vi "IP Cam Loop.vi"(11 "CameraDevRef":T1) -> ()   [LabVIEW 2015]
doc: "This VI acquires the image buffer from the camera MJPG stream at the configured fps rate. It notifies any waiting VIs and allows them to pick up the latest image. This allows the camera and robot vision loop to run at different rates. The 1011, camera is far more efficient using MJPGs, and generally, this is probably the better choice for the camera loop.\n \nThis software is licensed. Open the labview\\readme\\WPI Robotics Library Open Source License.txt file for more information."
uses:
  <vilib>/Rock Robotics/WPI/Camera/WPI_CameraDevRef.ctl
  <vilib>/Rock Robotics/WPI/Camera/WPI_CameraSettings Operations.ctl
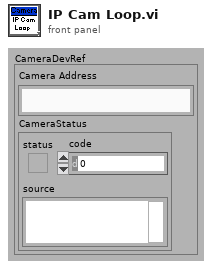
[diagram p1: front panel]
types:
  T1 = typedef "WPI_CameraDevRef.ctl" = cluster{"Camera Address":string, "CameraStatus":errorcluster}
  T2 = typedef "WPI_CameraSettings Operations.ctl" = enum16{"Udate FPS", "Update Compression", "Update Size", "Update White Balance", "Update Brightness", "Update Sharpness", "Update Exposure", "Update Exposure Value", "Update Color Level", "Update Exp Priority", "Update Color Enable", "Update JPG", "Update MJPG", "Read and Clear", "Read", "Init"}
  T3 = typedef "WPI_CameraSettings Control.ctl" = cluster{"FPS":i32, "Compression":i32, "Size":i32, "White Balance":i32, "Brightness":i32, "Sharpness":i32, "Exposure":i32, "Color Level":i32, "Exposure Priority":i32, "Color Enable":i32, "JPG Loop":i32, "MJPG Loop":i32, "Exposure Value":i32}
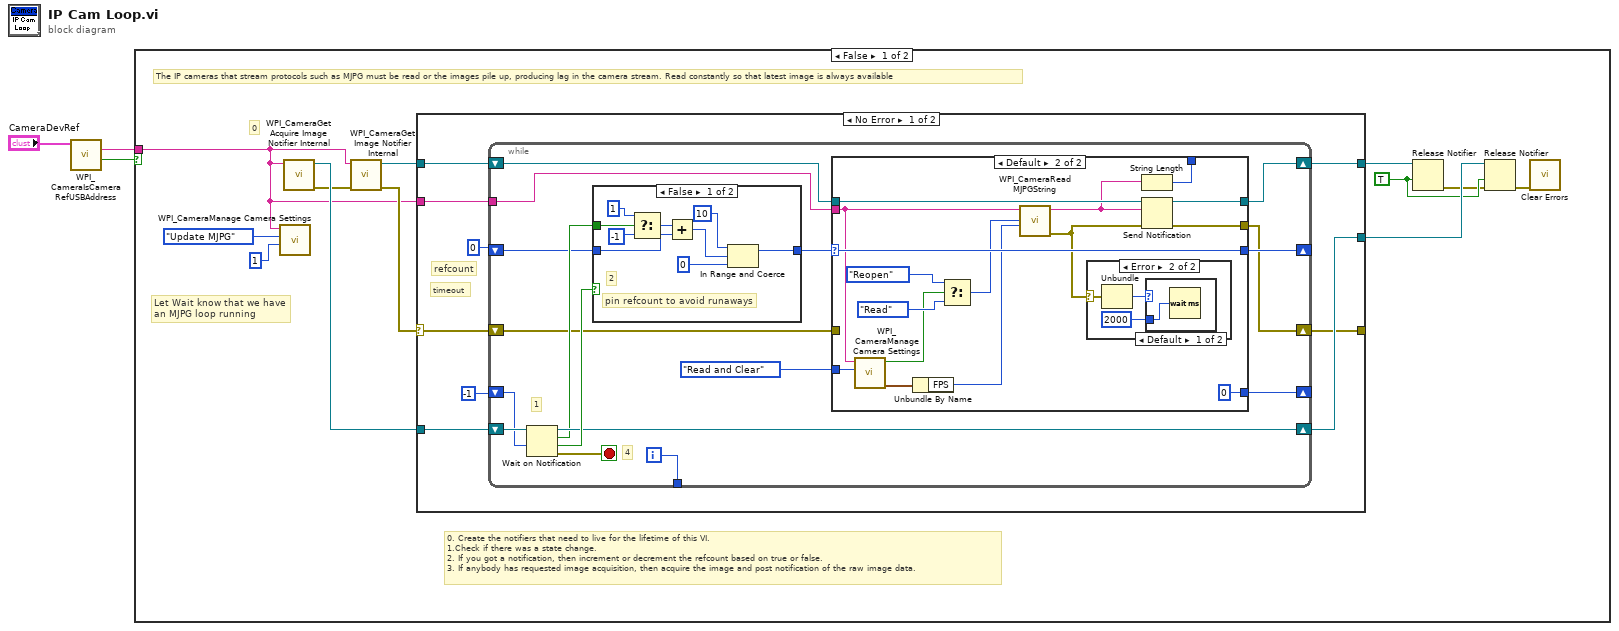
[diagram p0: block diagram]
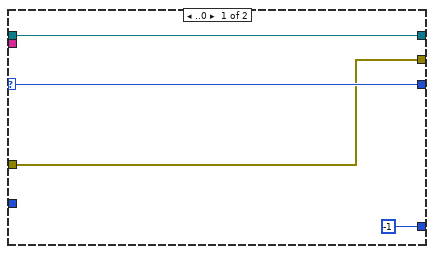
[diagram p2: hidden frame]
diagram:
  n1 = call <vilib>:"WPI_CameraIsCameraRefUSBAddress.vi"("CameraDevRef"="CameraDevRef") -> ("USB?"=w2:bool, "Camera Address Out"=w1:string)  [unwired: 7 in, 2 out]
  n2 = case shown="False" w2 {
    tunnel: w1 -> [w5 _]
    frame False {
      w12 = TRUE ("force destroy? (F)")
      # "The IP cameras that stream protocols such as MJPG must be read or the images pile up, producing lag in the camera stream. Read constantly so that latest image is always available"
      # "0. Create the notifiers that need to live for the lifetime of this VI. \n1.Check if there was a state change.\n2. If you got a notification, then increment or decrement the refcount based on true or false.\n3. If anybody has requested image acquisition, then acquire the image and post notification of the raw image data."
      # "Let Wait know that we have\nan MJPG loop running"
      # "0"
      n3 = call <vilib>:"WPI_CameraManage Camera Settings.vi"("Value"=1, "Operation"=WPI_CameraSettings_Operations."Update MJPG", "Camera IP"=w5) -> ()  [unwired: 7 in, 2 out]
      n4 = call <vilib>:"WPI_CameraGet Acquire Image Notifier Internal.vi"("Camera Address"=w5) -> ("error out"=w9:errorcluster, "Acquire Image Notifier"=w10:refnum<notifier>)  [unwired: 1 in, 8 out]
      n5 = call <vilib>:"WPI_CameraGet Image Notifier Internal.vi"("error in (no error)"=w9, "Camera Address"=w5) -> ("error out"=w11:errorcluster, "Image Notifier"=w13:refnum<notifier>)  [unwired: 8 out]
      n6 = case shown="No Error" w11 {
        selector: w11 -> [w17 w78]
        tunnel: w5 -> [w24 _]
        tunnel: w10 -> [w23 w76]
        tunnel: w13 -> [w21 w77]
        tunnel: [w19 w77] -> w15
        tunnel: [w18 w76] -> w14
        tunnel: [w16 w78] -> _
        frame No Error {
          # "timeout"
          # "refcount"
          n7 = while {
            shift-right: [w39] -> w18
            shift-left: w23 -> [w41]
            tunnel: w24 -> [w36]
            shift-right: [w28] -> _
            shift-left: 0 -> [w37]
            shift-right: [w34] -> w19
            shift-left: w21 -> [w35]
            shift-right: [w32] -> _
            shift-left: -1 -> [w33]
            shift-right: [w27] -> w16
            shift-left: w17 -> [w30]
            tunnel: [w25] -> _
            i -> [w25]
            stop <- w31 stop-if-true
            # "4"
            # "1"
            n8 = Wait on Notification(notifier=w41, timeout in ms (-1)=w33) -> (notifier out=w39:refnum<notifier>, notification=w38:bool, timed out?=w40:bool, error out=w31:errorcluster)  [unwired: 1 in, 1 out]
            n9 = case shown="False" w40 {
              tunnel: w38 -> [w74 _]
              tunnel: w37 -> [w70 w75]
              tunnel: [w66 w75] -> w29
              frame False {
                # "pin refcount to avoid runaways"
                # "2"
                n10 = Select(t=1, s=w74, f=-1) -> (s? t:f=w71:i32)
                n11 = Add(x=w71, y=w70) -> (x+y=w67:i32)
                n12 = In Range and Coerce(upper limit=10, x=w67, lower limit=0) -> (coerced(x)=w66:i32)  [unwired: 1 out]
              }
              frame True {
              }
            }
            n13 = case shown="Default" w29 {
              selector: w29 -> [w44 w58]
              tunnel: w36 -> [_ w46]
              tunnel: w35 -> [w45 w61]
              tunnel: [w45 w60] -> w34
              tunnel: [-1 0] -> w32
              tunnel: w30 -> [w42 _]
              tunnel: [w44 w58] -> w28
              tunnel: [w42 w57] -> w27
              tunnel: [_ w51] -> _
              tunnel: WPI_CameraSettings_Operations."Read and Clear" ("Operation") -> [_ w47]
              frame ..0 {
              }
              frame Default {
                n14 = call <vilib>:"WPI_CameraManage Camera Settings.vi"("Operation"=w47, "Camera IP"=w46) -> ("Values"=w49:T3, "Changed"=w50:bool)  [unwired: 8 in]
                n15 = Unbundle By Name(w49) -> ("FPS"=w48:i32)
                n16 = Select(t=enum16{"Read", "Reopen", "Close"}."Reopen" ("Operation"), s=w50, f=enum16{"Read", "Reopen", "Close"}."Read" ("Operation")) -> (s? t:f=w53:enum16{"Read", "Reopen", "Close"})
                n17 = call <vilib>:"WPI_CameraRead MJPGString.vi"("fps"=w48, "Operation"=w53, "address"=w46) -> ("error out"=w56:errorcluster, "Raw Image Data"=w52:string)  [unwired: 7 in]
                n18 = case shown="Error" w56 {
                  selector: w56 -> [_ w64]
                  frame No Error {
                  }
                  frame Error {
                    n19 = Unbundle(w64) -> ("code"=w63:i32)  [unwired: 2 out]
                    n20 = case shown="Default" w63 {
                      tunnel: u32 2000 ("milliseconds to wait") -> [w65 _]
                      frame Default {
                        n21 = Wait (ms)(milliseconds to wait=w65) -> ()  [unwired: 1 out]
                      }
                      frame 56 {
                      }
                    }
                  }
                }
                n22 = String Length(string=w52) -> (length=w51:i32)
                n23 = Send Notification(notification=w52, notifier=w61, error in (no error)=w56) -> (notifier out=w60:refnum<notifier>, error out=w57:errorcluster)
              }
            }
          }
        }
        frame Error {
        }
      }
      n24 = Release Notifier(notifier=w15, force destroy? (F)=w12) -> (error out=w8:errorcluster)  [unwired: 1 in, 2 out]
      n25 = Release Notifier(notifier=w14, force destroy? (F)=w12, error in (no error)=w8) -> (error out=w4:errorcluster)  [unwired: 2 out]
      n26 = call <vilib>:"Clear Errors.vi"("error in (no error)"=w4) -> ()  [unwired: 1 in, 6 out]
    }
    frame True {
      # "The USB cameras may need to be forwarded over ethernet. Read, compress, and send to the Dashbd."
    }
  }
